vi "0x16MaskPresetSingleRegister.vi"(6 "AndMask":u16 format="%.0x", 7 "ORMask":u16 format="%.0x", 8 "error in (no error)":errorcluster, 9 "Register":u16, 10 "Addressc":u8, 11 "ASCII in":refnum<class "ASCII.lvclass">) -> (0 "error out":errorcluster, 2 "Frame":string, 3 "ASCII out":refnum<class "ASCII.lvclass">)   [LabVIEW 2015, in "ModBUS.lvlib" / "ASCII.lvclass"]
uses:
  ASCII.lvclass
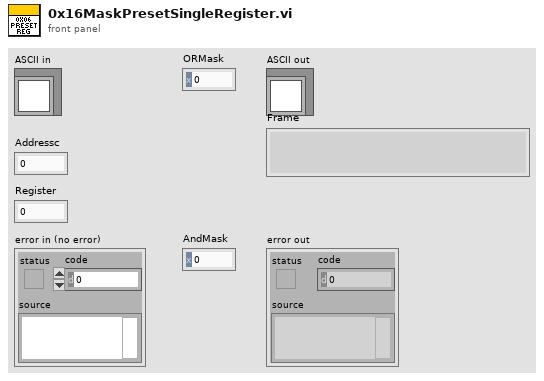
[diagram p1: front panel]
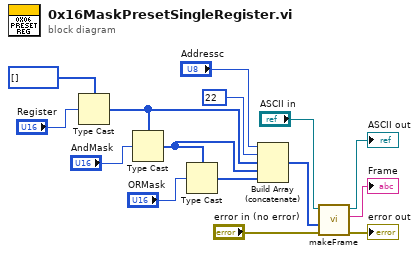
[diagram p0: block diagram]
diagram:
  n1 = Type Cast(type=u8[] [], x="Register") -> (*(type *) &x=w10:u8[])
  n2 = Type Cast(type=w10, x="AndMask") -> (*(type *) &x=w5:u8[])
  n3 = Type Cast(type=w5, x="ORMask") -> (*(type *) &x=w4:u8[])
  n4 = Build Array (concatenate)("Addressc", u8 22 ("element"), w10, w5, w4) -> (w1:u8[])
  n5 = call-dynamic "makeFrame.vi"("error in (no error)"="error in (no error)", "Data"=w1, "ASCII in"="ASCII in") -> ("error out"=→"error out":errorcluster, "Frame"=→"Frame":string, "ASCII out"=→"ASCII out":refnum<class "ASCII.lvclass">)  [unwired: 6 in]
